vi "alu.vi"(3 "Func":T2, 4 "B":T3, 5 "A":T4) -> (0 "S1":bool, 1 "Type":bool, 2 "R":T1)   [LabVIEW 2013]
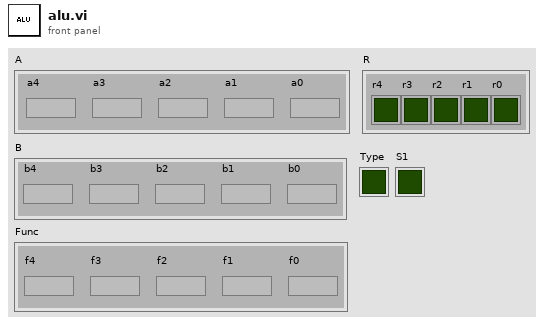
[diagram p1: front panel]
types:
  T1 = cluster{"r4":bool, "r3":bool, "r2":bool, "r1":bool, "r0":bool}
  T2 = cluster{"f4":bool, "f3":bool, "f2":bool, "f1":bool, "f0":bool}
  T3 = cluster{"b4":bool, "b3":bool, "b2":bool, "b1":bool, "b0":bool}
  T4 = cluster{"a4":bool, "a3":bool, "a2":bool, "a1":bool, "a0":bool}
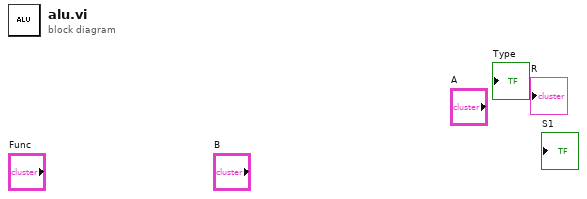
[diagram p0: block diagram]
diagram:
